vi "Write objChnls.vi"(8 "error in (no error)":errorcluster, 10 "objChnls":refnum<class "BME_DG_Chnl.lvclass">[](array[class])=[refnum, refnum, refnum], 11 "BME_DG_Base in":refnum<class "BME_DG_Base.lvclass">) -> (0 "error out":errorcluster, 3 "BME_DG_Base out":refnum<class "BME_DG_Base.lvclass">)   [LabVIEW 2009, in "BME_DG_Base.lvclass"]
uses:
  BME_DG_Base.lvclass
  BME_DG_Chnl/BME_DG_Chnl.lvclass
  BME_DG_Base.lvclass/BME_DG_Base.ctl
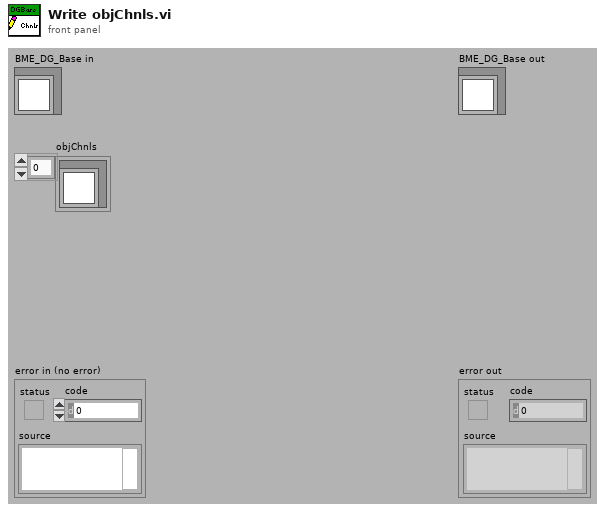
[diagram p1: front panel]
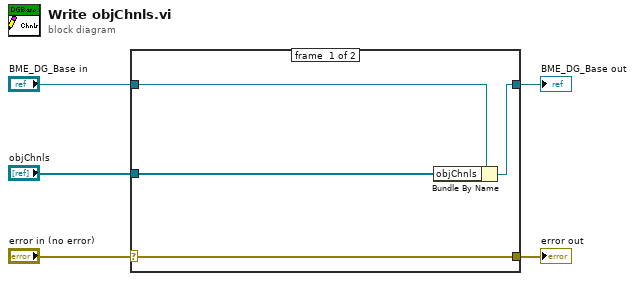
[diagram p0: block diagram]
diagram:
  n1 = case shown="No Error" "error in (no error)" {
    selector: "error in (no error)" -> [w9 w10]
    tunnel: [w9 w10] -> w4
    tunnel: [w7 w11] -> w2
    tunnel: "BME_DG_Base in" -> [w8 w11]
    tunnel: "objChnls" -> [w6 _]
    frame #0 {
      n2 = Bundle By Name(cluster=w8, "objChnls"=w6) -> (w7:refnum<class "BME_DG_Base.lvclass">)
    }
    frame #1 {
    }
  }
  "error out" <- w4
  "BME_DG_Base out" <- w2
